vi "TCP Discoverable Test Client.vi"() -> ()   [LabVIEW 2020]
panel:
  out "address":string
  out "error":errorcluster
  in  "Port":i32=4900
  in  "Command":string
  in  "Send":bool
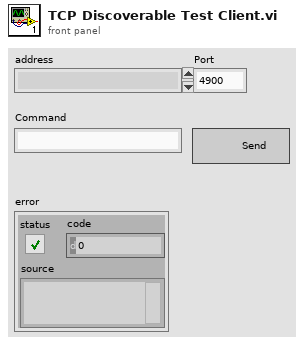
[diagram p1: front panel]
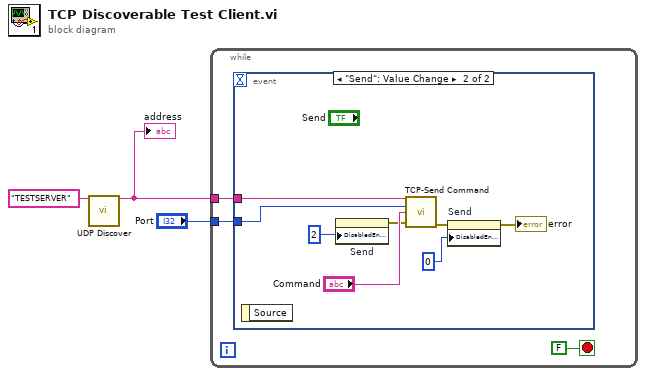
[diagram p0: block diagram]
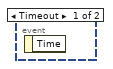
[diagram p2: hidden frame]
diagram:
  n1 = call "UDP Discover.vi"("Name"="TESTSERVER") -> ("address"=w2:string)  [unwired: 13 in, 1 out]
  "address" <- w2
  n2 = while {
    tunnel: w2 -> [w6]
    tunnel: "Port" -> [w5]
    stop <- FALSE stop-if-true
    n3 = event shown="[1] \"Send\": Value Change" {
      selector: _ -> [_ _]
      dyn-events: _ -> [_ _]
      timeout: _ -> [_ _]
      tunnel: w6 -> [_ w14]
      tunnel: w5 -> [_ w13]
      event Timeout {
        n4 = event-data() -> ()  [unwired: 1 in, 1 out]
      }
      event "Send": Value Change {
        n5 = event-data() -> ()  [unwired: 1 in, 1 out]
        n6 = property on="Send" class="Bool"("DisabledEnum"=2) -> (error out=w11:errorcluster)  [unwired: 2 in, 1 out]
        n7 = call "TCP-Send Command.vi"("PXI Address"=w14, "Port"=w13, "Command"="Command", "error in (no error)"=w11) -> ("error out"=w9:errorcluster)  [unwired: 11 in]
        n8 = property on="Send" class="Bool"(error in=w9, "DisabledEnum"=0) -> (error out=→"error":errorcluster)  [unwired: 1 in, 1 out]
      }
    }
  }
